vi "Update Connection.vi"(8 "error in":errorcluster, 11 "TCP Data":T1) -> (0 "error out":errorcluster)   [LabVIEW 2015]
uses:
  TCP/TypeDefs/TCP Data.ctl
  Message Queue/Message Queue.lvlib
  TCP/TCP.lvlib
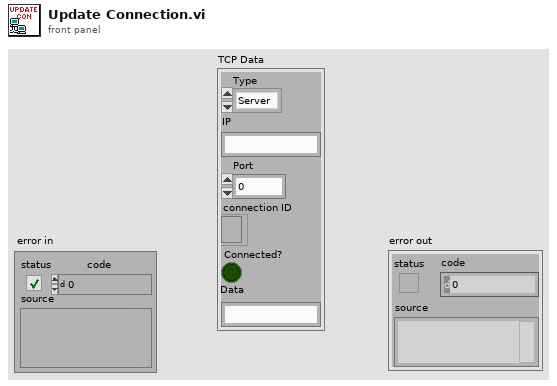
[diagram p1: front panel]
types:
  T1 = typedef "TCP.lvlib/TCP Data.ctl" = cluster{"Type":enum16{"Server", "Client"}, "IP":string, "Port":u16, "connection ID":refnum<k5>, "Connected?":bool, "Data":string}
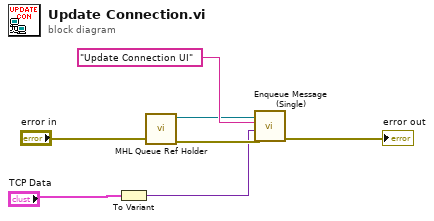
[diagram p0: block diagram]
diagram:
  n1 = To Variant(anything="TCP Data") -> (Variant=w2:variant)
  n2 = call "MHL Queue Ref Holder.vi"("error in"="error in") -> ("error out"=w3:errorcluster, "Input Message Queue"=w4:refnum<queue>)  [unwired: 9 in]
  n3 = call "Enqueue Message (Single).vi"("error in (no error)"=w3, "Message Data"=w2, "Message"="Update Connection UI", "Message Queue"=w4) -> ("error out"=→"error out":errorcluster)  [unwired: 6 in, 1 out]
